vi "Initialise Front Panel.vi"(7 "This VI":refnum<vi>, 11 "UI Ref":T1) -> (0 "error out":errorcluster)   [LabVIEW 2021]
uses:
  Controls/UI References.ctl
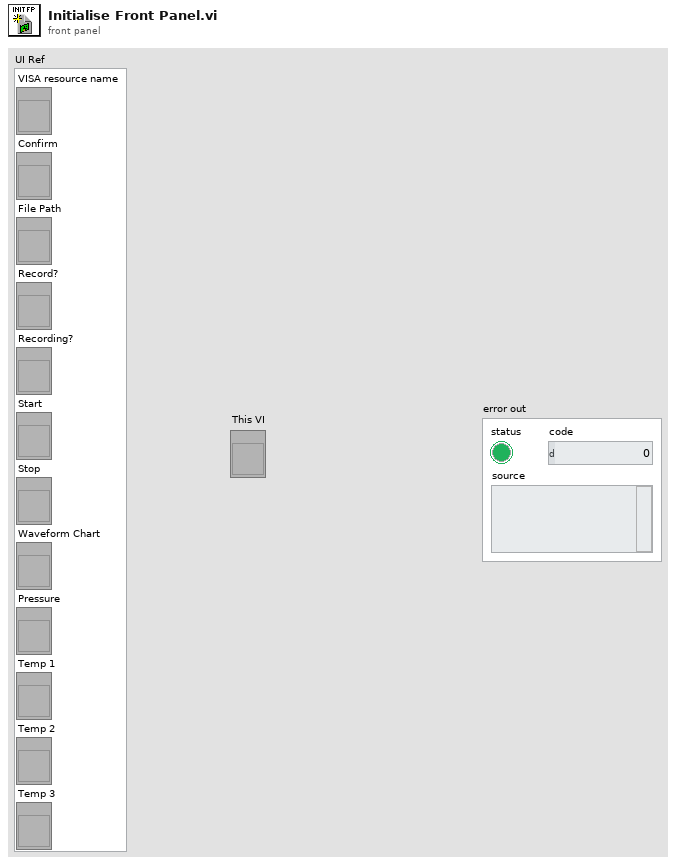
[diagram p1: front panel]
types:
  T1 = typedef "UI References.ctl" = cluster{"VISA resource name":refnum<vi>, "Confirm":refnum<vi>, "File Path":refnum<vi>, "Record?":refnum<vi>, "Recording?":refnum<vi>, "Start":refnum<vi>, "Stop":refnum<vi>, "Waveform Chart":refnum<vi>, "Pressure":refnum<vi>, "Temp 1":refnum<vi>, "Temp 2":refnum<vi>, "Temp 3":refnum<vi>}
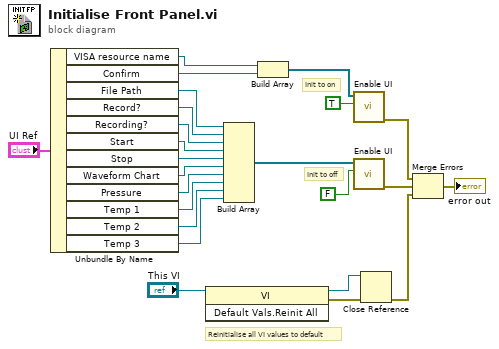
[diagram p0: block diagram]
diagram:
  # "Init to on"
  # "Init to off"
  # "Reinitialise all VI values to default"
  n1 = Unbundle By Name("UI Ref") -> ("VISA resource name"=w21:refnum<vi>, "Confirm"=w20:refnum<vi>, "File Path"=w17:refnum<vi>, "Record?"=w16:refnum<vi>, "Recording?"=w15:refnum<vi>, "Start"=w14:refnum<vi>, "Stop"=w13:refnum<vi>, "Waveform Chart"=w12:refnum<vi>, "Pressure"=w11:refnum<vi>, "Temp 1"=w10:refnum<vi>, "Temp 2"=w9:refnum<vi>, "Temp 3"=w8:refnum<vi>)
  n2 = invoke class="VI" method="Default Vals.Reinit All"(reference="This VI") -> (reference out=w22:refnum<vi>, error out=w5:errorcluster)  [unwired: 2 in, 1 out]
  n3 = Build Array(w17, w16, w15, w14, w13, w12, w11, w10, w9, w8) -> (w7:refnum<vi>[])
  n4 = Build Array(w21, w20) -> (w19:refnum<vi>[])
  n5 = call "Enable UI.vi"("Enable?"=TRUE, "output cluster"=w19) -> ("error out"=w4:errorcluster)  [unwired: 9 in]
  n6 = call "Enable UI.vi"("Enable?"=FALSE, "output cluster"=w7) -> ("error out"=w3:errorcluster)  [unwired: 9 in]
  n7 = Close Reference(reference=w22, error in (no error)=w5) -> (error out=w2:errorcluster)
  n8 = Merge Errors(w4, w3, w2) -> (→"error out":errorcluster)
